vi "Type.vi"(11 "Type in":refnum<class "Type.lvclass">) -> (2 "Type":T1)   [LabVIEW 2020, in "Conditum.lvlib" / "Columns.lvlib" / "Type.lvclass"]
uses:
  Type.lvclass
  LabVIEW Type.ctl
  Conditum.lvlib
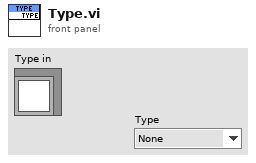
[diagram p1: front panel]
types:
  T1 = typedef "Conditum.lvlib/LabVIEW Type.ctl" = enum16{"None", "ID", "Boolean", "Integer", "Double", "Timestamp", "String", "Text", "Entity"}
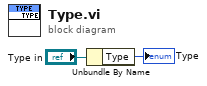
[diagram p0: block diagram]
diagram:
  n1 = Unbundle By Name("Type in") -> ("Type"=→"Type":T1)
